vi "WriteDM_V2.vi"(0 "reference in":refnum<k7>, 1 "nDevId":i32, 2 "MultiDM  Mapping":i32[](array[numeric]), 3 "Voltage Array in":dbl[](array[numeric]), 4 "error in":errorcluster) -> (5 "reference out":refnum<k7>, 7 "error out":errorcluster)   [LabVIEW 2014]
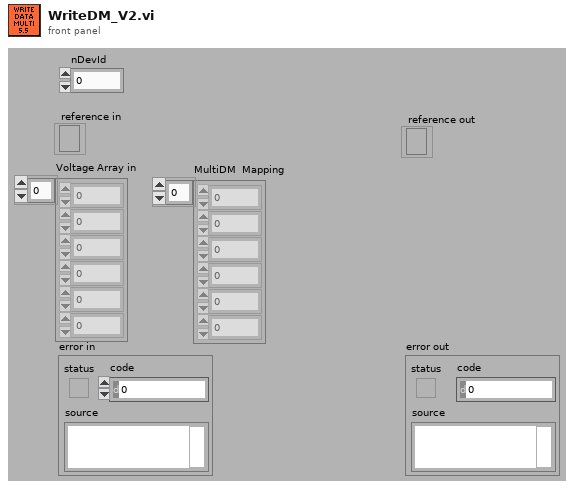
[diagram p1: front panel]
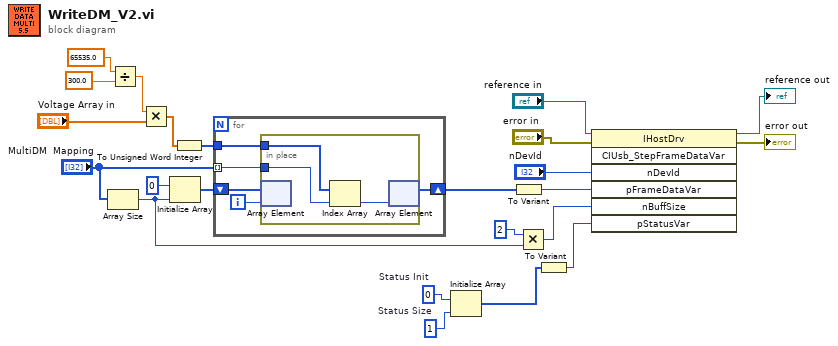
[diagram p0: block diagram]
diagram:
  w9 = 1  # Status Size
  w8 = 0  # Status Init
  n1 = Array Size(array="MultiDM  Mapping") -> (size(s)=w4:i32)
  n2 = Divide(x=65535.0 ("y"), y=300.0 ("x")) -> (x/y=w5:dbl)
  n3 = Multiply(x=w5, y="Voltage Array in") -> (x*y=w18:dbl[])
  n4 = Initialize Array(u16 0 ("element"), w4) -> (w16:u16[])
  n5 = To Unsigned Word Integer(number=w18) -> (unsigned 16bit integer=w14:u16[])
  n6 = for {
    shift-right: [w26] -> w13
    shift-left: w16 -> [w28]
    tunnel: "MultiDM  Mapping" -> [w24] mode=indexing
    tunnel: w14 -> [w27]
    i -> [w25]
    n7 = in-place {
      in-place-border: w27 -> [w30]
      in-place-border: w24 -> [w31]
      n8 = in-place-array #1(w28, w25) -> ()  [unwired: 1 out]
      n9 = Index Array(array=w30, index=w31) -> (element=w29:u16)
      n10 = in-place-array #1(w29) -> (w26:u16[])  [unwired: 1 out]
    }
  }
  n11 = Initialize Array "Initialize Array"(w8, w9) -> (w7:i32[])
  n12 = To Variant(anything=w13) -> (Variant=w21:variant)
  n13 = Multiply(x=2, y=w4) -> (x*y=w2:i32)
  n14 = To Variant(anything=w7) -> (Variant=w6:variant)
  n15 = invoke class="IHostDrv" method="CIUsb_StepFrameDataVar"(reference="reference in", error in="error in", "nDevId"="nDevId", "pFrameDataVar"=w21, "nBuffSize"=w2, "pStatusVar"=w6) -> (reference out=→"reference out":refnum<k7>, error out=→"error out":errorcluster)  [unwired: 1 in, 5 out]
